vi "Main.vi"(11 "Module Admin":refnum<class "Delacor_lib_QMH_Module Admin.lvclass">) -> ()   [LabVIEW 2023, in "UDP RT.lvlib"]
doc: "This template is based off of the Queued Message Handler design pattern and the Queued Message Handler project template that ships with LabVIEW.\n\nThe main difference is that the queue is private to this module and communication between modules is performed via Broadcast and Request events.\n\nRequest events are wrapped in public API methods and are handled in the Event Handling Loop (EHL) of this VI. Any module can register for Broadcast events sent by this module. The EHL generates messages based on user interface actions.\n\nThe Message Handling Loop (MHL) processes messages generated by the EHL, or by other messages. The messages are string values, so new messages can be added easily to the Message Cases case structure in the MHL. Each message cluster can also provide an optional value for Message Data, which is a variant that can be converted to whatever message-specific data is required.\n_____\nBased on DQMH Dev Tools: Project Template 7.1.2.1547."
uses:
  UDP RT.lvlib
  <vilib>/Delacor/Delacor QMH/Libraries/Module Admin_class/Delacor_lib_QMH_Module Admin.lvclass
  Module Data--cluster.ctl
  Stop Argument--cluster.ctl
  <vilib>/Delacor/Delacor QMH/Libraries/Message Queue_class/Delacor_lib_QMH_Message Queue.lvclass/Delacor_lib_QMH_Message Queue.ctl
  <vilib>/Delacor/Delacor QMH/Libraries/Module Admin_class/Delacor_lib_QMH_Module Admin.lvclass/Delacor_lib_QMH_Module Admin.ctl
  <vilib>/Delacor/Delacor QMH/Libraries/Message Queue_class/Delacor_lib_QMH_Enqueue Message (Single).vi
  <vilib>/Delacor/Delacor QMH/Libraries/Module Admin_class/Delacor_lib_QMH_Get External Launch.vi
  <vilib>/Delacor/Delacor QMH/Libraries/Message Queue_class/Delacor_lib_QMH_Message Queue.lvclass
panel:
  out "error out":errorcluster
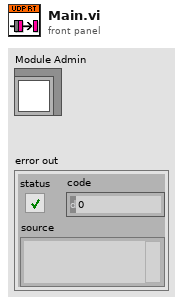
[diagram p1: front panel]
types:
  T1 = typedef "UDP RT.lvlib/Request Events--cluster.ctl" = cluster{"Stop Module":refnum<user-event>, "Show Panel":refnum<user-event>, "Hide Panel":refnum<user-event>, "Get Module Execution Status":refnum<user-event>, "Show Diagram":refnum<user-event>, "Private.Open Connection":refnum<user-event>}
  T2 = typedef "UDP RT.lvlib/Module Data--cluster.ctl" = cluster{"IP Host":string, "Port RT":u16, "Port Host":u16, "connection ID":refnum<k16>}
  T3 = enum32{"invalid lock state", "Not Locked", "Locked (No Password)", "Password-protected"}
  T4 = typedef "UDP RT.lvlib/Stop Argument--cluster.ctl" = cluster{"Origin":string, "Exit via Stop Module Req?":bool, "Wait for Module to stop?":bool}
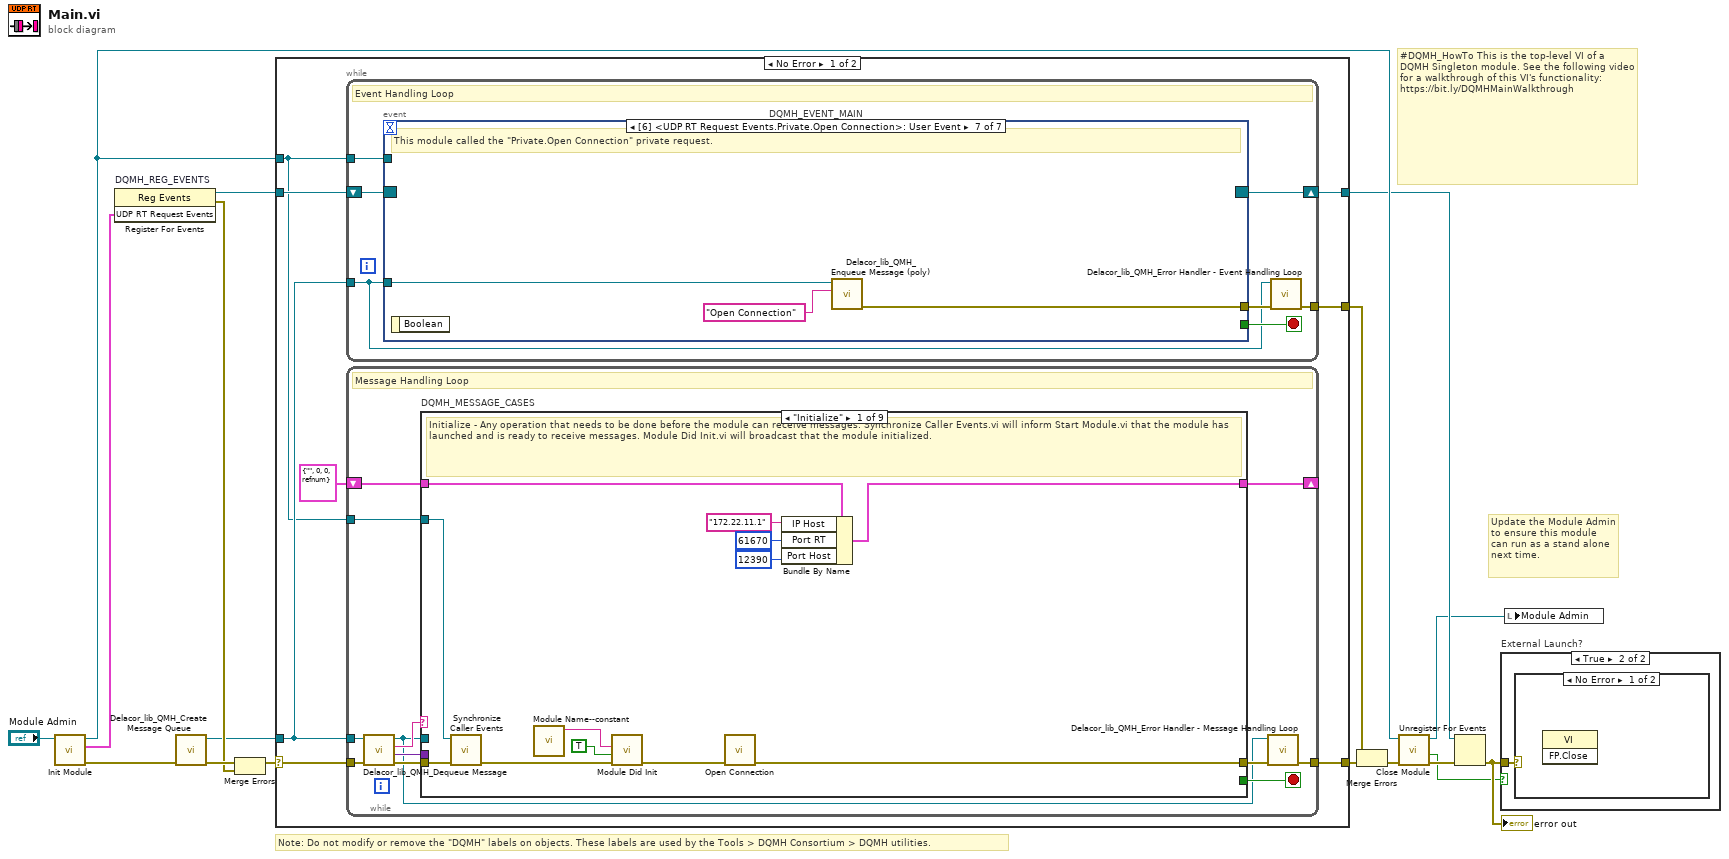
[diagram p0: block diagram]
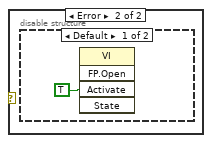
[diagram p3: hidden frame]
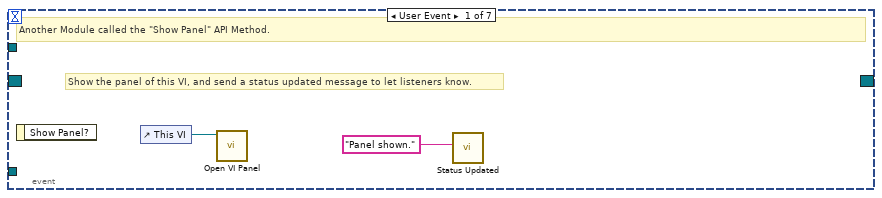
[diagram p5: hidden frame]
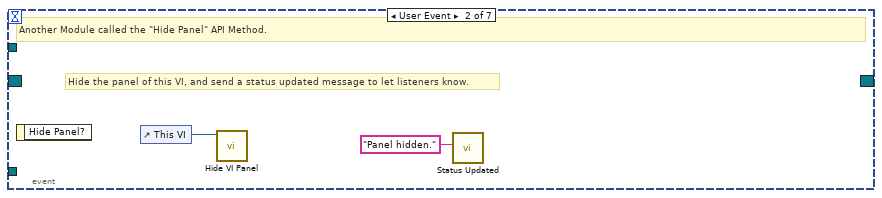
[diagram p6: hidden frame]
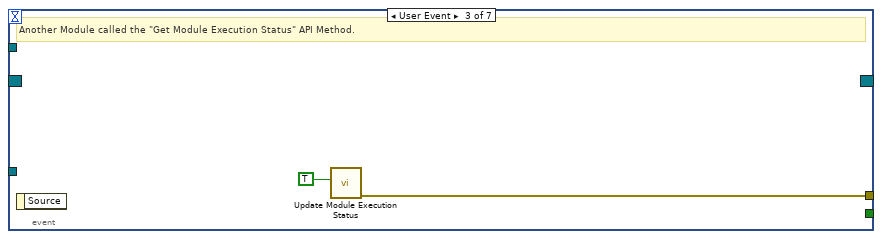
[diagram p7: hidden frame]
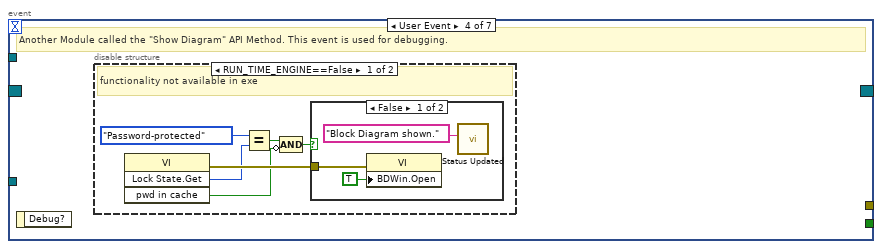
[diagram p8: hidden frame]
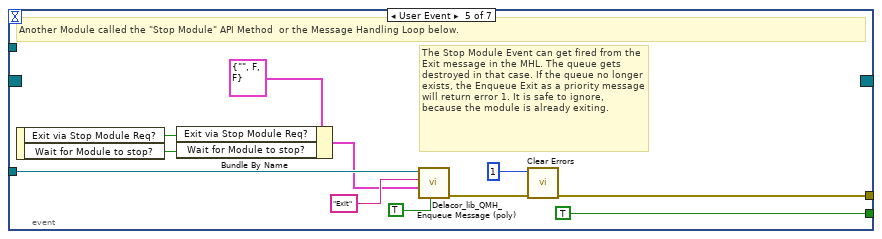
[diagram p11: hidden frame]
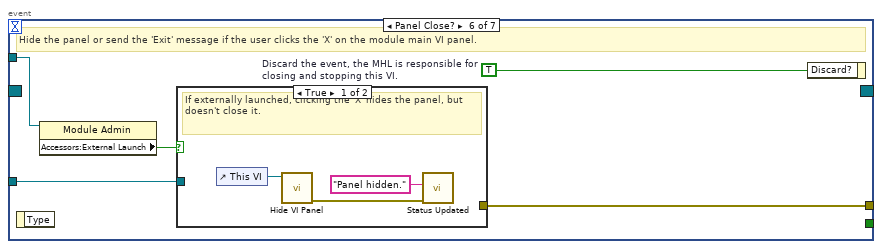
[diagram p12: hidden frame]
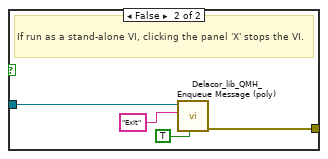
[diagram p13: hidden frame]
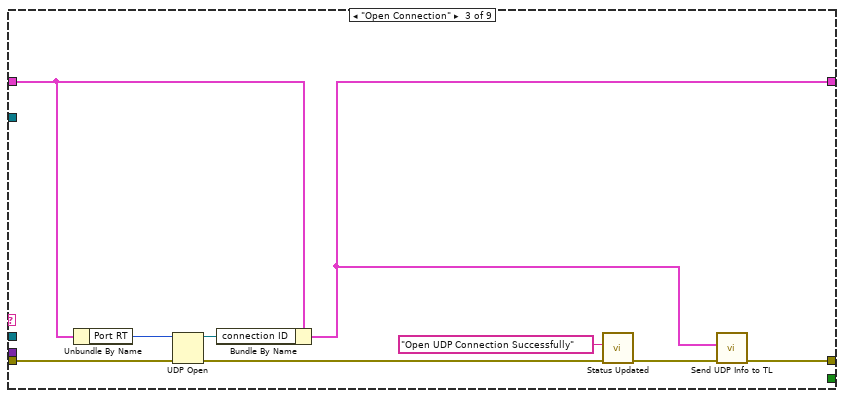
[diagram p15: hidden frame]
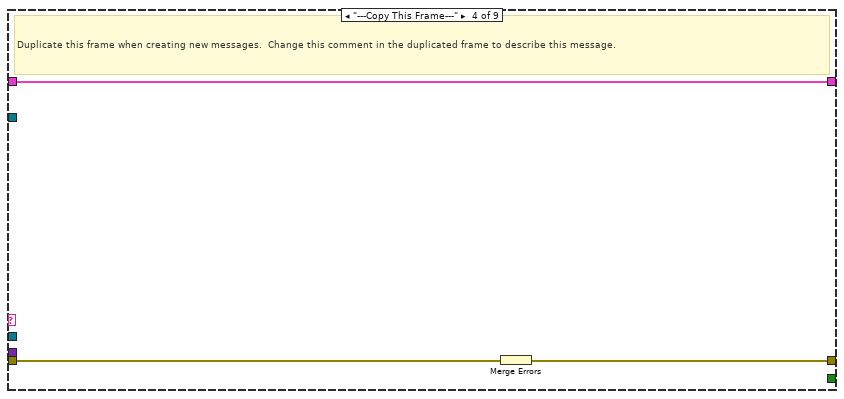
[diagram p16: hidden frame]
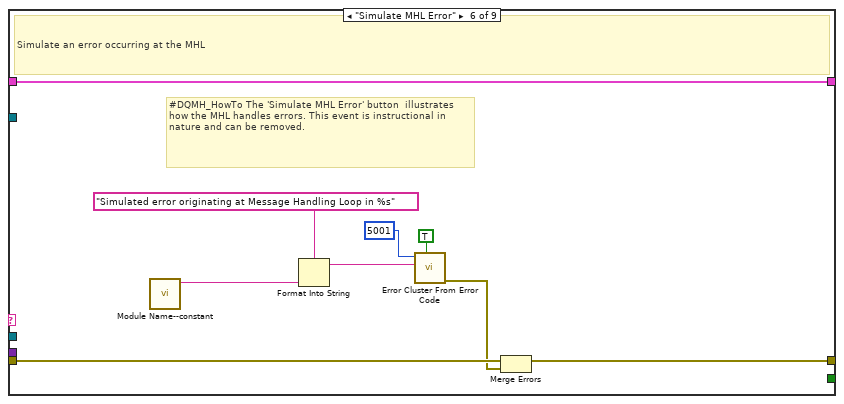
[diagram p18: hidden frame]
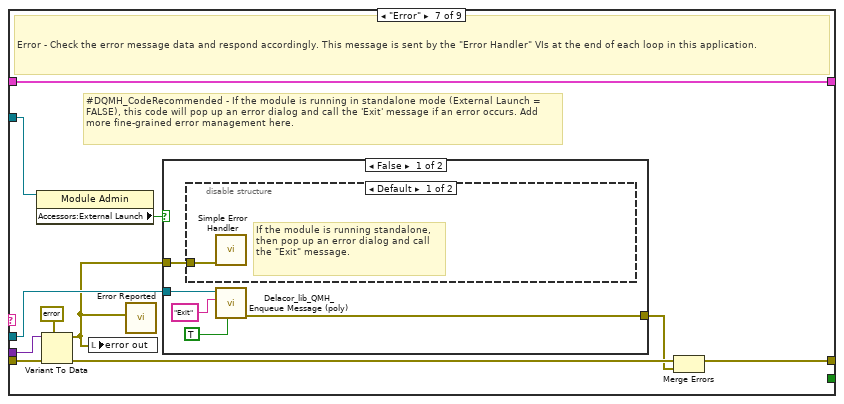
[diagram p19: hidden frame]
diagram:
  # "#DQMH_HowTo This is the top-level VI of a DQMH Singleton module. See the following video for a walkthrough of this VI's functionality: https://bit.ly/DQMHMainWalkthrough"
  # "Note: Do not modify or remove the \"DQMH\" labels on objects. These labels are used by the Tools > DQMH Consortium > DQMH utilities."
  # "Update the Module Admin to ensure this module can run as a stand alone next time."
  n1 = call "Init Module.vi"("Singleton Module Admin in"="Module Admin") -> ("error out"=w16:errorcluster, "UDP RT Request Events"=w5:T1, "Singleton Module Admin out"=w8:refnum<class "Delacor_lib_QMH_Module Admin.lvclass">)  [unwired: 8 in]
  n2 = register-events "DQMH_REG_EVENTS"(w5) -> (reference out=w6:refnum<event-registration>, error out=w9:errorcluster)  [unwired: 2 in]
  n3 = call <vilib>:"Delacor_lib_QMH_Create Message Queue.vi"("error in"=w16) -> ("error out"=w11:errorcluster, "Message Queue"=w4:refnum<class "Delacor_lib_QMH_Message Queue.lvclass">)  [unwired: 9 in]
  n4 = Merge Errors(w11, w9) -> (w10:errorcluster)
  n5 = case shown="No Error" w10 {
    selector: w10 -> [w23 w173]
    tunnel: [w25 w172] -> w17
    tunnel: [w22 w171] -> w7
    tunnel: w6 -> [w20 w171]
    tunnel: w4 -> [w19 w166]
    tunnel: [w24 _] -> w14
    tunnel: w8 -> [w18 w167]
    frame No Error {
      n6 = while {
        tunnel: w19 -> [w26]
        shift-right: [w29] -> w22
        shift-left: w20 -> [w30]
        tunnel: [w31] -> w24
        tunnel: w18 -> [w27]
        stop <- w28 stop-if-true
        # "Event Handling Loop"
        n7 = event "DQMH_EVENT_MAIN" shown="[6] <UDP RT Request Events.Private.Open Connection>: User Event" {
          selector: w30 -> [_ _ _ _ _ _ _]
          dyn-events: [_ _ _ _ _ _ _] -> w29
          timeout: _ -> [_ _ _ _ _ _ _]
          tunnel: [_ _ _ _ TRUE ("Discard?") _ _] -> w28
          tunnel: w26 -> [_ _ _ _ w54 w61 w73]
          tunnel: [_ _ w38 _ w57 w63 w71] -> w32
          tunnel: w27 -> [_ _ _ _ _ w60 _]
          event User Event {
            # "Show the panel of this VI, and send a status updated message to let listeners know."
            # "Another Module called the \"Show Panel\" API Method."
            n8 = event-data() -> ()  [unwired: 1 in, 1 out]
            n9 = control-ref of="This VI"() -> (w34:refnum<vi>)
            n10 = call "Open VI Panel.vi"("VI"=w34) -> ()  [unwired: 10 in, 1 out]
            n11 = call "Status Updated.vi"("Status"="Panel shown." ("format string")) -> ()  [unwired: 10 in, 1 out]
          }
          event User Event {
            # "Hide the panel of this VI, and send a status updated message to let listeners know."
            # "Another Module called the \"Hide Panel\" API Method."
            n12 = event-data() -> ()  [unwired: 1 in, 1 out]
            n13 = control-ref of="This VI"() -> (w36:refnum<vi>)
            n14 = call "Hide VI Panel.vi"("VI"=w36) -> ()  [unwired: 10 in, 1 out]
            n15 = call "Status Updated.vi"("Status"="Panel hidden." ("format string")) -> ()  [unwired: 10 in, 1 out]
          }
          event User Event {
            # "Another Module called the \"Get Module Execution Status\" API Method."
            n16 = event-data() -> ()  [unwired: 1 in, 1 out]
            n17 = call "Update Module Execution Status.vi"("Running?"=TRUE) -> ("error out"=w38:errorcluster)  [unwired: 10 in]
          }
          event User Event {
            # "Another Module called the \"Show Diagram\" API Method. This event is used for debugging."
            n18 = event-data() -> ()  [unwired: 1 in, 1 out]
            n19 = disable-structure shown="RUN_TIME_ENGINE==False" {
              frame condition #0 (active) {
                # "functionality not available in exe"
                n20 = invoke on="Invoke Node" class="VI" method="Lock State.Get"() -> (error out=w44:errorcluster, "Get Lock State"=w43:T3, "pwd in cache"=w40:bool)  [unwired: 4 in, 1 out]
                n21 = Equal?(x=T3."Password-protected", y=w43) -> (x = y?=w41:bool)
                n22 = Compound Arithmetic op=AND(w41, invert w40) -> (w39:bool)
                n23 = case shown="False" w39 {
                  tunnel: w44 -> [w47 _]
                  frame False {
                    n24 = property on="Property Node" class="VI"(error in=w47, "BDWin.Open"=TRUE ("Block Diagram Window:Open")) -> ()  [unwired: 1 in, 2 out]
                    n25 = call "Status Updated.vi"("Status"="Block Diagram shown." ("format string")) -> ()  [unwired: 10 in, 1 out]
                  }
                  frame True {
                    # "Password-protected VI, and the password is not in the cache. Do not show the diagram."
                  }
                }
              }
              frame condition #1 {
              }
            }
          }
          event User Event {
            # "The Stop Module Event can get fired from the Exit message in the MHL. The queue gets destroyed in that case. If the queue no longer exists, the Enqueue Exit as a priority message will return error 1. It is safe to ignore, because the module is already exiting."
            # "Another Module called the \"Stop Module\" API Method  or the Message Handling Loop below."
            n26 = event-data() -> ("Exit via Stop Module Req?"=w50:bool, "Wait for Module to stop?"=w49:bool)  [unwired: 1 in]
            n27 = Bundle By Name(cluster=T4 {"Origin"="", "Exit via Stop Module Req?"=FALSE, "Wait for Module to stop?"=FALSE} ("Stop Argument"), "Exit via Stop Module Req?"=w50, "Wait for Module to stop?"=w49) -> (w48:T4)
            n28 = call-poly <vilib>:"Delacor_lib_QMH_Enqueue Message (poly).vi"("Priority Message? (F)"=TRUE, "Message Data"=w48, "Message"="Exit", "Message Queue in"=w54) -> ("error out"=w58:errorcluster)  [unwired: 6 in, 1 out]
            n29 = call <vilib>:"Clear Errors.vi"("error in (no error)"=w58, "specific error code to clear (0: all)"=1) -> ("error out"=w57:errorcluster)  [unwired: 4 in, 1 out]
          }
          event Panel Close? {
            w62 = TRUE  # Discard the event, the MHL is responsible for closing and stopping this VI.
            # "Hide the panel or send the 'Exit' message if the user clicks the 'X' on the module main VI panel."
            n30 = event-data() -> ()  [unwired: 1 in, 1 out]
            n31 = property on="Property Node" class="Module Admin"(reference=w60) -> ("Accessors:External Launch"=w59:bool)  [unwired: 1 in, 2 out]
            n32 = case shown="True" w59 {
              tunnel: w61 -> [_ w69]
              tunnel: [_ w70] -> w63
              frame True {
                # "If externally launched, clicking the 'X' hides the panel, but doesn't close it."
                n33 = control-ref of="This VI"() -> (w66:refnum<vi>)
                n34 = call "Hide VI Panel.vi"("VI"=w66) -> ("error out"=w64:errorcluster)  [unwired: 10 in]
                n35 = call "Status Updated.vi"("error in"=w64, "Status"="Panel hidden." ("format string")) -> ()  [unwired: 9 in, 1 out]
              }
              frame False {
                # "If run as a stand-alone VI, clicking the panel 'X' stops the VI."
                n36 = call-poly <vilib>:"Delacor_lib_QMH_Enqueue Message (poly).vi"("Priority Message? (F)"=TRUE, "Message"="Exit", "Message Queue in"=w69) -> ("error out"=w70:errorcluster)  [unwired: 7 in, 1 out]
              }
            }
            n37 = event-data ("Event Filter Node")("Discard?"=w62) -> ()  [unwired: 1 in, 1 out]
          }
          event User Event {
            # "This module called the \"Private.Open Connection\" private request."
            n38 = event-data() -> ()  [unwired: 1 in, 1 out]
            n39 = call-poly <vilib>:"Delacor_lib_QMH_Enqueue Message (poly).vi"("Message"="Open Connection", "Message Queue in"=w73) -> ("error out"=w71:errorcluster)  [unwired: 8 in, 1 out]
          }
        }
        n40 = call-dynamic "Delacor_lib_QMH_Error Handler - Event Handling Loop.vi"("error in"=w32, "Message Queue in"=w26) -> ("dup error in"=w31:errorcluster)  [unwired: 8 in, 1 out]
      }
      n41 = while {
        tunnel: w19 -> [w74]
        shift-right: [w82] -> _
        shift-left: T2 {"IP Host"="", "Port RT"=0, "Port Host"=0, "connection ID"=refnum} ("Data Cluster") -> [w83]
        tunnel: w23 -> [w85]
        tunnel: [w77] -> w25
        tunnel: w18 -> [w78]
        stop <- w81 stop-if-true
        # "Message Handling Loop"
        n42 = call-dynamic "Delacor_lib_QMH_Dequeue Message.vi"("error in"=w85, "Message Queue in"=w74) -> ("error out"=w84:errorcluster, "Message Data"=w79:variant, "Message"=w80:string, "Message Queue out"=w75:refnum<class "Delacor_lib_QMH_Message Queue.lvclass">)  [unwired: 6 in]
        n43 = case "DQMH_MESSAGE_CASES" shown="\"Initialize\"" w80 {
          selector: w80 -> [_ _ _ _ _ _ _ _ w161]
          tunnel: w75 -> [_ _ _ _ _ _ w126 w149 _]
          tunnel: w84 -> [w97 w99 w108 w111 w113 w122 w133 w155 w164]
          tunnel: [w91 w99 w101 w110 w113 w121 w129 w150 w165] -> w76
          tunnel: w83 -> [w89 w98 w104 w109 w112 w119 w128 w141 w162]
          tunnel: [w90 w98 w100 w109 w112 w119 w128 w141 w162] -> w82
          tunnel: [_ _ _ _ _ _ _ w148 _] -> w81
          tunnel: w79 -> [_ _ _ _ _ _ w127 w147 _]
          tunnel: w78 -> [w95 _ _ _ _ _ w125 w142 _]
          frame "Initialize" {
            # "Initialize - Any operation that needs to be done before the module can receive messages. Synchronize Caller Events.vi will inform Start Module.vi that the module has launched and is ready to receive messages. Module Did Init.vi will broadcast that the module initialized."
            n44 = call "Synchronize Caller Events.vi"("error in"=w97, "Singleton Module Admin in"=w95) -> ("error out"=w96:errorcluster)  [unwired: 8 in, 1 out]
            n45 = call "Module Name--constant.vi"() -> ("Module Name"=w93:string)  [unwired: 11 in]
            n46 = call "Module Did Init.vi"("error in"=w96, "Initialized?"=TRUE, "Origin"=w93) -> ("error out"=w92:errorcluster)  [unwired: 8 in]
            n47 = call "Open Connection.vi"("error in"=w92) -> ("error out"=w91:errorcluster)  [unwired: 10 in]
            n48 = Bundle By Name(cluster=w89, "IP Host"="172.22.11.1", "Port RT"=u16 61670, "Port Host"=u16 12390) -> (w90:T2)
          }
          frame "---Module Specific---" {
            # "Separator -- The following cases handle messages specific to this Module."
          }
          frame "Open Connection" {
            n49 = Unbundle By Name(w104) -> ("Port RT"=w103:u16)
            n50 = UDP Open(8:w108, 11:w103) -> (port=w107:refnum<k16>, 0:w106:errorcluster)  [unwired: 3 in, 1 out]
            n51 = Bundle By Name(cluster=w104, "connection ID"=w107) -> (w100:T2)
            n52 = call "Status Updated.vi"("error in"=w106, "Status"="Open UDP Connection Successfully") -> ("error out"=w102:errorcluster)  [unwired: 9 in]
            n53 = call "Send UDP Info to TL.vi"("error in"=w102, "UDP Info"=w100) -> ("error out"=w101:errorcluster)  [unwired: 9 in]
          }
          frame "---Copy This Frame---" {
            # "Duplicate this frame when creating new messages.  Change this comment in the duplicated frame to describe this message."
            n54 = Merge Errors(w111) -> (w110:errorcluster)
          }
          frame "---Exit and Error Handling---" {
            # "Separator - The following cases handle errors and exit messages."
          }
          frame "Simulate MHL Error" {
            # "#DQMH_HowTo The 'Simulate MHL Error' button  illustrates how the MHL handles errors. This event is instructional in nature and can be removed."
            # "Simulate an error occurring at the MHL"
            n55 = call "Module Name--constant.vi"() -> ("Module Name"=w115:string)  [unwired: 11 in]
            n56 = Format Into String(format string="Simulated error originating at Message Handling Loop in %s", w115) -> (resulting string=w116:string)  [unwired: 2 in, 1 out]
            n57 = call <vilib>:"Error Cluster From Error Code.vi"("show call chain? (False)"=TRUE, "error message (\"\")"=w116, "error code (0)"=5001) -> ("error out"=w120:errorcluster)  [unwired: 6 in]
            n58 = Merge Errors(w122, w120) -> (w121:errorcluster)
          }
          frame "Error" {
            # "#DQMH_CodeRecommended - If the module is running in standalone mode (External Launch = FALSE), this code will pop up an error dialog and call the 'Exit' message if an error occurs. Add more fine-grained error management here."
            # "Error - Check the error message data and respond accordingly. This message is sent by the \"Error Handler\" VIs at the end of each loop in this application."
            n59 = property on="Property Node" class="Module Admin"(reference=w125) -> ("Accessors:External Launch"=w124:bool)  [unwired: 1 in, 2 out]
            n60 = Variant To Data(error in=w133, type=errorcluster {"status"=FALSE, "code"=0, "source"=""} ("error constant"), Variant=w127) -> (data=w123:errorcluster, error out=w131:errorcluster)
            n61 = local write "error out"(w123) -> ()
            n62 = call "Error Reported.vi"("Error"=w123) -> ()  [unwired: 10 in, 1 out]
            n63 = case shown="False" w124 {
              tunnel: [w138 _] -> w130
              tunnel: w126 -> [w136 _]
              tunnel: w123 -> [w137 _]
              frame False {
                n64 = disable-structure shown="Default" {
                  disable-tunnel: w137 -> [w139 _]
                  frame condition #0 (active) {
                    # "If the module is running standalone, then pop up an error dialog and call the \"Exit\" message."
                    n65 = call <vilib>:"Simple Error Handler.vi"("error in (no error)"=w139) -> ()  [unwired: 4 in, 5 out]
                  }
                  frame condition #1 {
                    # "To prevent the Simple Error Handler VI from being loaded (e.g. when deploying to a Real-Time target), add the Conditional Disable Symbol \"DQMH_Disable_SEH\" to your project and set it to TRUE."
                  }
                }
                n66 = call-poly <vilib>:"Delacor_lib_QMH_Enqueue Message (poly).vi"("Priority Message? (F)"=TRUE, "Message"="Exit", "Message Queue in"=w136) -> ("error out"=w138:errorcluster)  [unwired: 7 in, 1 out]
              }
              frame True {
                # "If the module was launched externally, calling the Error Reported broadcast VI is the only action performed by the \"Error\" message. The module's caller can then process the error appropriately."
              }
            }
            n67 = Merge Errors(w131, w130) -> (w129:errorcluster)
          }
          frame "Exit" {
            w146 = 91  # 91: not all Exit messages will have an argument
            w148 = TRUE  # Stop the VI
            # "Release the message queue reference"
            # "Exit - Exit the application."
            n68 = Variant To Data(error in=w155, type=T4 {"Origin"="", "Exit via Stop Module Req?"=FALSE, "Wait for Module to stop?"=FALSE} ("Stop Argument"), Variant=w147) -> (data=w144:T4, error out=w152:errorcluster)
            n69 = call <vilib>:"Clear Errors.vi"("error in (no error)"=w152, "specific error code to clear (0: all)"=w146) -> ("error out"=w154:errorcluster)  [unwired: 4 in, 1 out]
            n70 = control-ref of="This VI"() -> (w143:refnum<vi>)
            n71 = call-dynamic "Delacor_lib_QMH_Release Message Queue.vi"("error in"=w154, "Message Queue"=w149) -> ("error out"=w153:errorcluster)  [unwired: 9 in]
            n72 = call "Handle Exit.vi"("Stop Argument"=w144, "Admin in"=w142, "VI reference"=w143) -> ("error out"=w151:errorcluster)  [unwired: 7 in, 1 out]
            n73 = Merge Errors(w153, w151) -> (w150:errorcluster)
            n74 = Unbundle By Name(w141) -> ("connection ID"=w140:refnum<k16>)
            n75 = call "Error Reported.vi"("Error"=w150) -> ()  [unwired: 10 in, 1 out]
            n76 = UDP Close(connection ID=w140) -> ()  [unwired: 1 in, 2 out]
          }
          frame Default {
            # "'Default' case only runs if there is a message that isn't defined in any of the other cases.  Output a programming error."
            n77 = call "Module Name--constant.vi"() -> ("Module Name"=w160:string)  [unwired: 11 in]
            n78 = Format Into String(format string="The invalid message string \"%s\" was received in the Message Handling Loop for module \"%s\".", w161, w160) -> (resulting string=w156:string)  [unwired: 2 in, 1 out]
            n79 = call <vilib>:"Error Cluster From Error Code.vi"("show call chain? (False)"=TRUE, "error message (\"\")"=w156, "error code (0)"=1) -> ("error out"=w163:errorcluster)  [unwired: 6 in]
            n80 = Merge Errors(w164, w163) -> (w165:errorcluster)
          }
        }
        n81 = call-dynamic "Delacor_lib_QMH_Error Handler - Message Handling Loop.vi"("error in"=w76, "Message Queue in"=w75) -> ("dup error in"=w77:errorcluster)  [unwired: 8 in, 1 out]
      }
    }
    frame Error {
      # "Synchronize Caller Events.vi will inform Start Module.vi that the module has launched and will let the code calling Start Module.vi register for broadcasts and would permit the caller receive the broadcast that an error occurred at launch time."
      n82 = call-dynamic "Delacor_lib_QMH_Release Message Queue.vi"("error in"=w173, "Message Queue"=w166) -> ("error out"=w172:errorcluster)  [unwired: 9 in]
      n83 = call "Synchronize Caller Events.vi"("Singleton Module Admin in"=w167) -> ("error out"=w174:errorcluster)  [unwired: 9 in, 1 out]
      n84 = call "Module Name--constant.vi"() -> ("Module Name"=w170:string)  [unwired: 11 in]
      n85 = Format Into String(format string="An error occurred during initialization. %s is no longer running.", w170) -> (resulting string=w168:string)  [unwired: 2 in, 1 out]
      n86 = Merge Errors(w172, w174) -> (w175:errorcluster)
      n87 = call "Error Reported.vi"("Additional Information"=w168, "Error"=w175) -> ()  [unwired: 9 in, 1 out]
    }
  }
  n88 = Merge Errors(w14, w17) -> (w13:errorcluster)
  n89 = call "Close Module.vi"("error in"=w13, "Module Admin in"=w8) -> ("error out"=w15:errorcluster, "External Launch"=w1:bool, "Module Admin out"=w2:refnum<class "Delacor_lib_QMH_Module Admin.lvclass">)  [unwired: 7 in]
  n90 = Unregister For Events(event registration refnum=w7, error in=w15) -> (error out=w12:errorcluster)
  "error out" <- w12
  n91 = case "External Launch?" shown="True" w1 {
    tunnel: w12 -> [_ w176]
    frame False {
    }
    frame True {
      n92 = case shown="No Error" w176 {
        frame No Error {
          n93 = invoke on="Invoke Node" class="VI" method="FP.Close"() -> ()  [unwired: 3 in, 3 out]
        }
        frame Error {
          n94 = disable-structure shown="Default" {
            frame condition #0 (active) {
              n95 = invoke class="VI" method="FP.Open"("Activate"=TRUE ("Activate?")) -> ()  [unwired: 4 in, 5 out]
            }
            frame condition #1 {
              # "Don't show panel on error if running inside a built EXE."
            }
          }
        }
      }
    }
  }
  n96 = local write "Module Admin"(w2) -> ()
